vi "KEYSIGHT_DSO3034G_config.vi"() -> ()   [LabVIEW 2026]
panel:
  out "read buffer":string
  out "element":refnum<vi>
  out "All Objects[]":refnum<vi>[](array[refnum])
  out "Controls[]":refnum<vi>[](array[refnum])
  in  "Cluster":T1={"Boolean"=FALSE, "Boolean 2"=FALSE, "CH1"=-5.0}
  out "Array 2":string[](array[string])
  in  "Channel Scale":T2={"CH1"=2.1, "CH2"=2.0, "CH3"=2.0, "CH4"=2.0}
  out "Array":string[](array[string])
  in  "Channel offset":T2={"CH1"=-5.0, "CH2"=-1.0, "CH3"=3.0, "CH4"=7.0}
  in  "Channel enable":T3
  out "error out":errorcluster
  in  "write buffer":string=":DISPlay:DATA? PNG, COLOR"
  in  "VISA resource name":refnum<visa-resource-name>
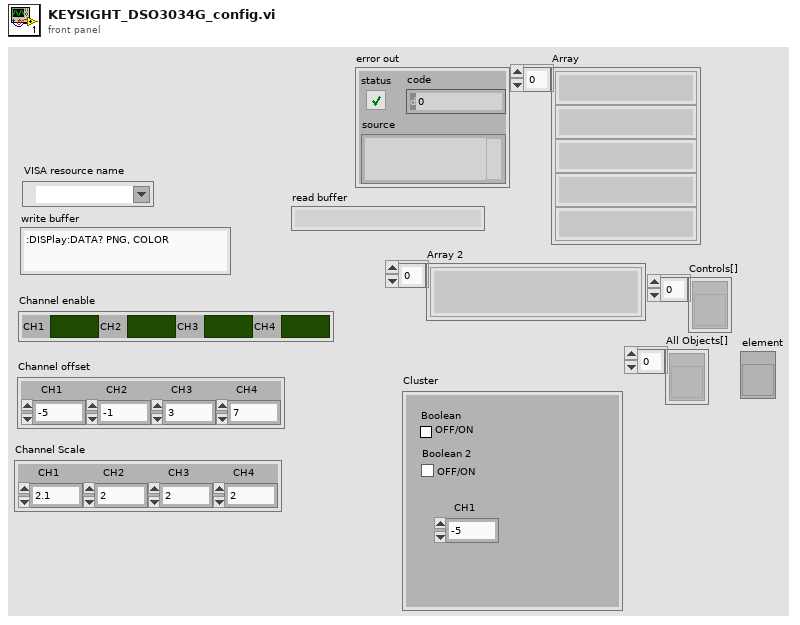
[diagram p1: front panel]
types:
  T1 = cluster{"Boolean":bool, "Boolean 2":bool, "CH1":dbl}
  T2 = cluster{"CH1":dbl, "CH2":dbl, "CH3":dbl, "CH4":dbl}
  T3 = cluster{"CH1":bool, "CH2":bool, "CH3":bool, "CH4":bool}
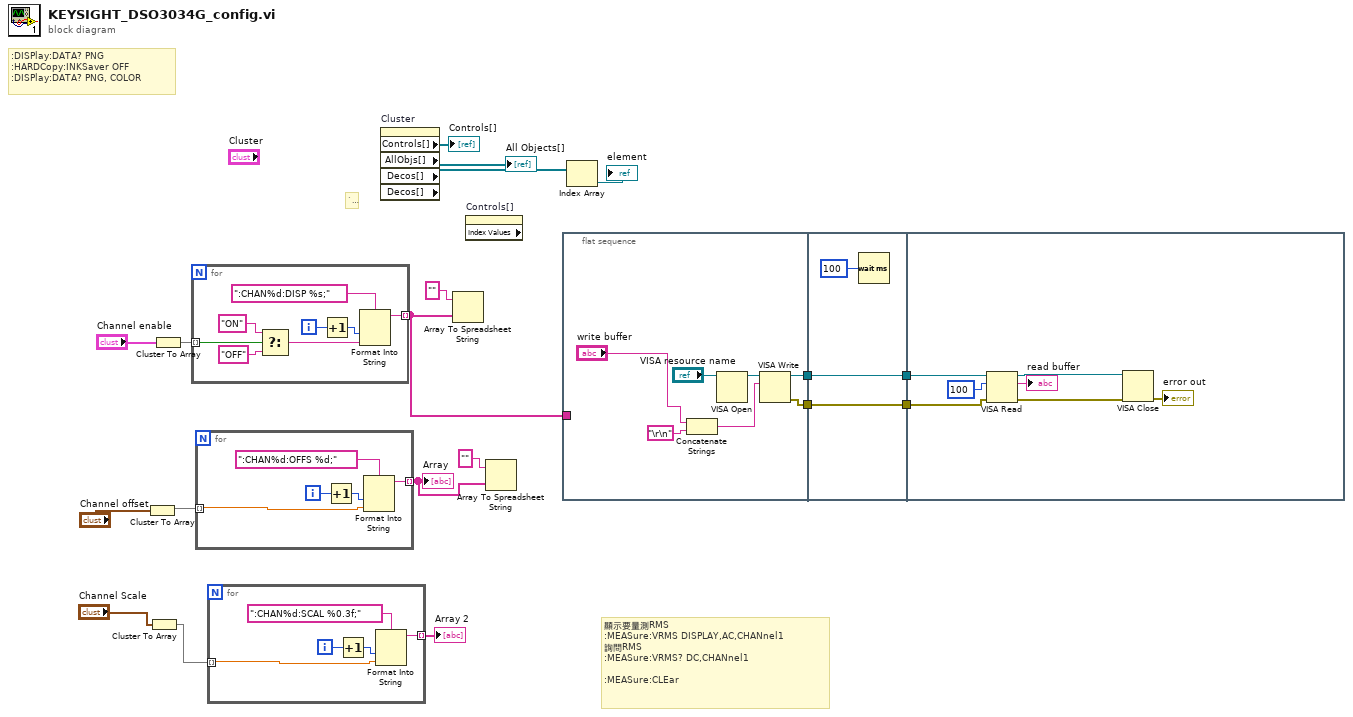
[diagram p0: block diagram]
diagram:
  # "顯示要量測RMS\n:MEASure:VRMS DISPLAY,AC,CHANnel1\n詢問RMS\n:MEASure:VRMS? DC,CHANnel1\n\n:MEASure:CLEar"
  # "```"
  # ":DISPlay:DATA? PNG\n:HARDCopy:INKSaver OFF\n:DISPlay:DATA? PNG, COLOR"
  n1 = Cluster To Array(cluster="Channel offset") -> (array=w10:dbl[])
  n2 = Cluster To Array(cluster="Channel Scale") -> (array=w6:dbl[])
  n3 = Cluster To Array(cluster="Channel enable") -> (array=w12:bool[])
  n4 = for {
    tunnel: w12 -> [w24] mode=indexing
    tunnel: [w21] -> w4 mode=indexing
    i -> [w20]
    n5 = Select(t="ON", s=w24, f="OFF") -> (s? t:f=w22:string)
    n6 = Increment(x=w20) -> (x+1=w19:i32)
    n7 = Format Into String(format string=":CHAN%d:DISP %s;", w19, w22) -> (resulting string=w21:string)  [unwired: 2 in, 1 out]
  }
  n8 = for {
    tunnel: w10 -> [w27] mode=indexing
    tunnel: [w30] -> w8 mode=indexing
    i -> [w29]
    n9 = Increment(x=w29) -> (x+1=w28:i32)
    n10 = Format Into String(format string=":CHAN%d:OFFS %d;", w28, w27) -> (resulting string=w30:string)  [unwired: 2 in, 1 out]
  }
  "Array" <- w8
  n11 = for {
    tunnel: w6 -> [w32] mode=indexing
    tunnel: [w35] -> w5 mode=indexing
    i -> [w34]
    n12 = Increment(x=w34) -> (x+1=w33:i32)
    n13 = Format Into String(format string=":CHAN%d:SCAL %0.3f;", w33, w32) -> (resulting string=w35:string)  [unwired: 2 in, 1 out]
  }
  "Array 2" <- w5
  n14 = property on="Cluster" class="Clust (strict)" props=["Controls[]", "AllObjs[]", "Decos[]", "Decos[]"]() -> ("Controls[]"=→"Controls[]":refnum<vi>[], "AllObjs[]"=w2:refnum<vi>[])  [unwired: 2 in, 4 out]
  "All Objects[]" <- w2
  n15 = Array To Spreadsheet String(array=w4, 3:"" ("format string")) -> ()  [unwired: 1 in, 1 out]
  n16 = property on="Controls[]" class="Arr (strict)" props=["Index Values"]() -> ()  [unwired: 2 in, 3 out]
  n17 = Array To Spreadsheet String(array=w8, 3:"" ("format string")) -> ()  [unwired: 1 in, 1 out]
  n18 = flat-sequence {
    tunnel: [w39] -> w18
    tunnel: [w38] -> w16
    tunnel: w4 -> [_]
    tunnel: w18 -> [w45]
    tunnel: [w45] -> w17
    tunnel: w16 -> [w44]
    tunnel: [w44] -> w15
    tunnel: w17 -> [w52]
    tunnel: w15 -> [w49]
    frame #0 {
      n19 = Concatenate Strings("write buffer", "\r\n") -> (w40:string)
      n20 = VISA Open(VISA resource name="VISA resource name") -> (VISA resource name=w42:refnum<visa-resource-name>)  [unwired: 4 in, 1 out]
      n21 = VISA Write(VISA resource name=w42, write buffer=w40) -> (VISA resource name out=w39:refnum<visa-resource-name>, error out=w38:errorcluster)  [unwired: 1 in, 1 out]
    }
    frame #1 {
      n22 = Wait (ms)(milliseconds to wait=u32 100) -> ()  [unwired: 1 out]
    }
    frame #2 {
      n23 = VISA Read(VISA resource name=w52, byte count=u32 100, error in (no error)=w49) -> (VISA resource name out=w51:refnum<visa-resource-name>, read buffer=→"read buffer":string, error out=w50:errorcluster)  [unwired: 1 out]
      n24 = VISA Close(VISA resource name=w51, error in (no error)=w50) -> (error out=→"error out":errorcluster)
    }
  }
  n25 = Index Array(array=w2) -> (element=→"element":refnum<vi>)  [unwired: 1 in]
